vi "mod_Create Continuous FSK (generic PN).vi"(0 "Filter Length":i32=8, 2 "Symbol Rate, Hz":dbl=1500000.0 format="%.2p", 4 "TX Filter":T1(ring), 6 "BT":dbl=0.5 format="%.2f", 7 "tolerance":dbl=1e-09, 8 "error in (no error)":errorcluster, 9 "bits per symbol":i32=1, 10 "PN Sequence Order":i32=9, 11 "FSK system parameters":T2={"samples per symbol (16)"=16, "symbol map"=[-650000.0, 650000.0], "symbol phase continuity"=enum."continuous"} {"symbol map" format="%.2p"}) -> (1 "error out":errorcluster={"status"=TRUE, "code"=-21816, "source"="mod_Create Continuous FSK (Bose).vi -> MT Generate Filter Coefficients.vi\r\n"}, 3 "samples per symbol":i32, 5 "output complex waveform":T3 {"Y" format="%.3f"; "dt" format="%^.2e"; "t0" format="%.4f"})   [LabVIEW 2020, in "niDMT.lvlib"]
uses:
  <vilib>/addons/Modulation/niDMT.lvlib
  <vilib>/addons/Modulation/Analog/controls/Complex Data Waveform.ctl
  <vilib>/addons/Modulation/Digital/Support/Controls/FSK System Parameters.ctl
  <vilib>/addons/Modulation/Digital/General/MT Generate Bits (Galois, PN Order).vi
  <vilib>/addons/Modulation/Digital/Support/Common/Validators/mod_Generate Bits Validate.vi
  <vilib>/addons/Modulation/Analog/support/mod_Set Error Source.vi
  <vilib>/addons/Modulation/Digital/Support/Common/Validators/mod_Generate Filter Coefficients Validate.vi
  <vilib>/addons/Modulation/Digital/General/subVIs/mod_Generate Filter Coefficients.vi
  <vilib>/addons/Modulation/Digital/General/subVIs/mod_Generate Bits PN Sequence.vi
  <vilib>/addons/Modulation/niAMT.lvlib
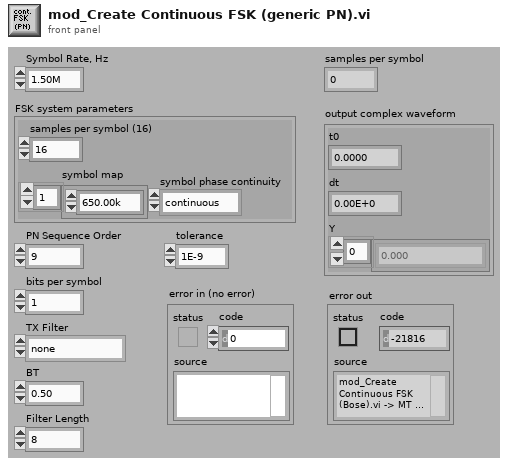
[diagram p1: front panel]
types:
  T1 = enum16{"none", "Raised Cosine", "Root Raised Cos", "Gaussian"}
  T2 = typedef "niDMT.lvlib/FSK System Parameters.ctl" = cluster{"samples per symbol (16)":i32, "symbol map":dbl[], "symbol phase continuity":enum16{"continuous", "discontinuous"}}
  T3 = typedef "niAMT.lvlib/Complex Data Waveform.ctl" = cluster{"t0":dbl, "dt":dbl, "Y":cdb[]}
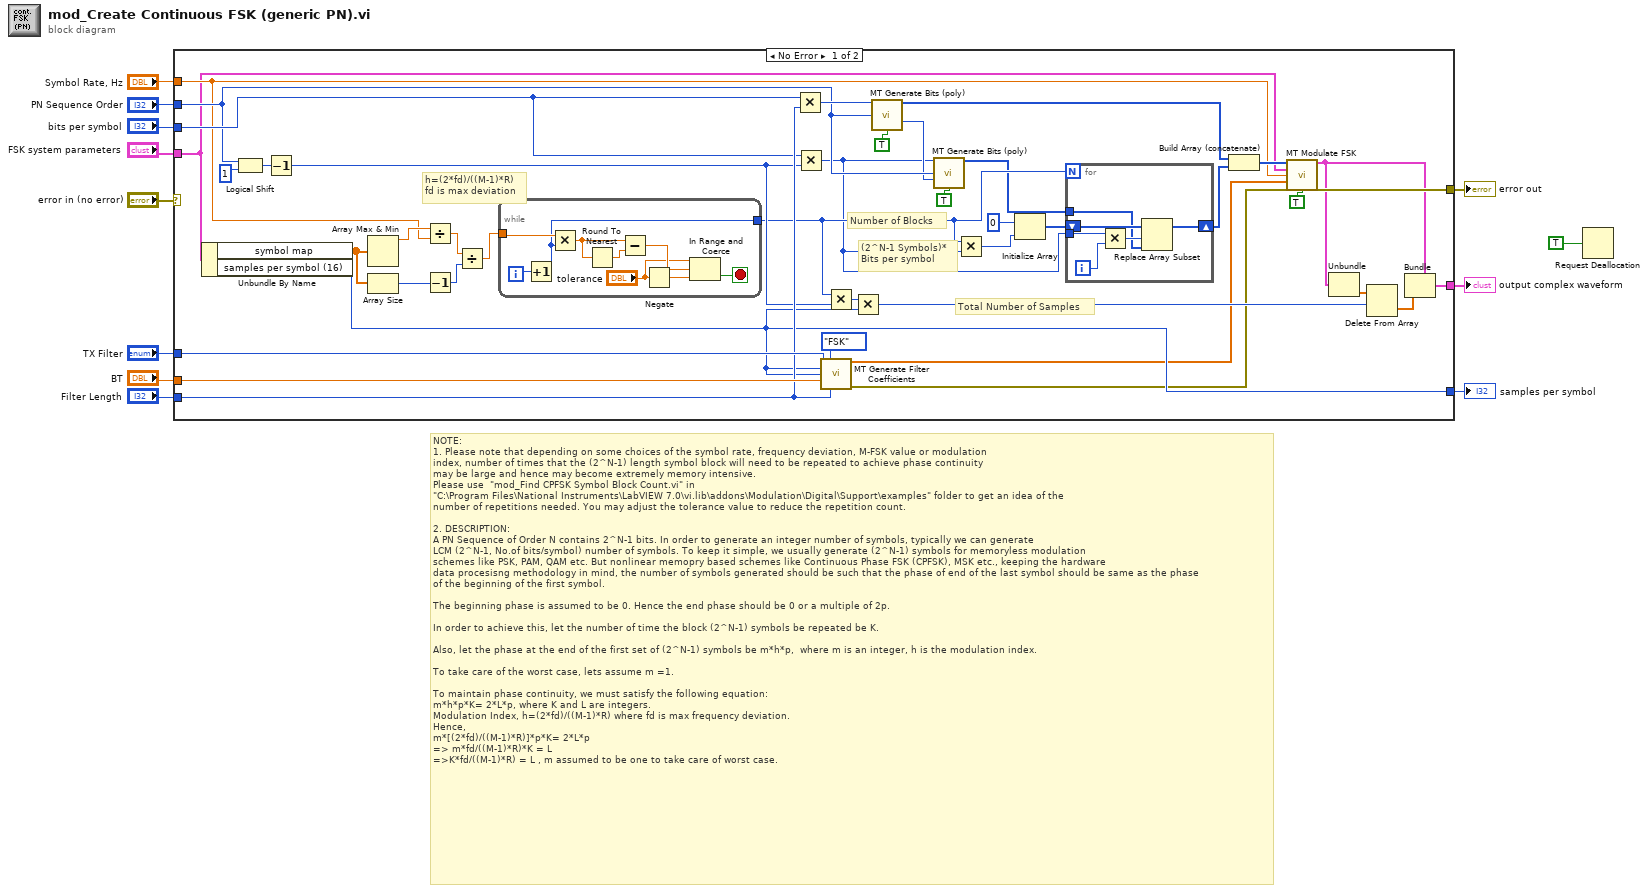
[diagram p0: block diagram]
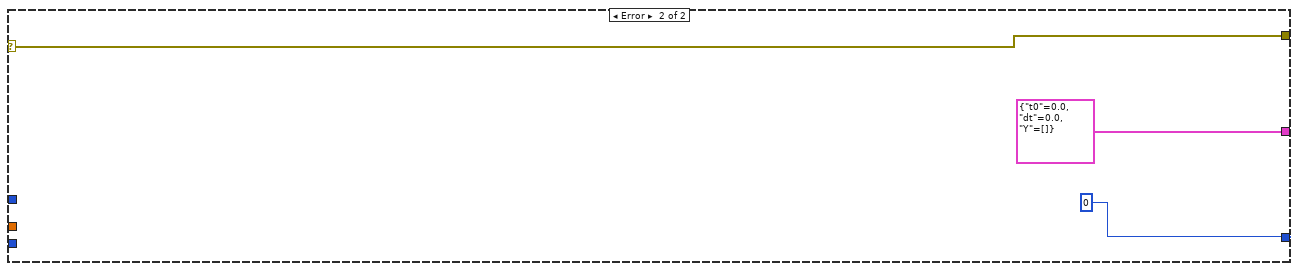
[diagram p2: hidden frame]
diagram:
  # "NOTE:\n1. Please note that depending on some choices of the symbol rate, frequency deviation, M-FSK value or modulation \nindex, number of times that the (2^N-1) length symbol block will need to be repeated to achieve phase continuity \nmay be large and hence may become extremely memory intensive. \nPlease use  \"mod_Find CPFSK Symbol Block Count.vi\" in  \n\"C:\\Program Files\\National Instruments\\LabVIEW 7.0\\vi.lib\\addons\\Modulation\\Digital\\Support\\examples\" folder to get an idea of the \nnumber of repetitions needed. You may adjust the tolerance value to reduce the repetition count.\n\n2. DESCRIPTION: \nA PN Sequence of Order N contains 2^N-1 bits. In order to generate an integer number of symbols, typically we can generate \nLCM (2^N-1, No.of bits/symbol) number of symbols. To keep it simple, we usually generate (2^N-1) symbols for memoryless modulation \nschemes like PSK, PAM, QAM etc. But nonlinear memopry based schemes like Continuous Phase FSK (CPFSK), MSK etc., keeping the hardware \ndata procesisng methodology in mind, the number of symbols generated should be such that the phase of end of the last symbol should be same as the phase \nof the beginning of the first symbol. \n\nThe beginning phase is assumed to be 0. Hence the end phase should be 0 or a multiple of 2p. \n\nIn order to achieve this, let the number of time the block (2^N-1) symbols be repeated be K. \n\nAlso, let the phase at the end of the first set of (2^N-1) symbols be m*h*p,  where m is an integer, h is the modulation index. \n\nTo take care of the worst case, lets assume m =1. \n\nTo maintain phase continuity, we must satisfy the following equation: \nm*h*p*K= 2*L*p, where K and L are integers. \nModulation Index, h=(2*fd)/((M-1)*R) where fd is max frequency deviation. \nHence, \nm*[(2*fd)/((M-1)*R)]*p*K= 2*L*p \n=> m*fd/((M-1)*R)*K = L \n=>K*fd/((M-1)*R) = L , m assumed to be one to take care of worst case."
  n1 = case shown="No Error" "error in (no error)" {
    selector: "error in (no error)" -> [_ w69]
    tunnel: [w53 w69] -> w12
    tunnel: [w52 cluster{"t0":dbl, "dt":dbl, "Y":cdb[]} {"t0"=0.0, "dt"=0.0, "Y"=[]} ("output complex waveform")] -> w10
    tunnel: [w31 0 ("samples per symbol (16)")] -> w9
    tunnel: "Symbol Rate, Hz" -> [w16 _]
    tunnel: "PN Sequence Order" -> [w24 _]
    tunnel: "bits per symbol" -> [w25 _]
    tunnel: "FSK system parameters" -> [w15 _]
    tunnel: "TX Filter" -> [w38 _]
    tunnel: "BT" -> [w37 _]
    tunnel: "Filter Length" -> [w36 _]
    frame No Error {
      # "Total Number of Samples"
      # "Number of Blocks"
      # "(2^N-1 Symbols)*\nBits per symbol"
      # "h=(2*fd)/((M-1)*R)\nfd is max deviation"
      n2 = Unbundle By Name(w15) -> ("symbol map"=w30:dbl[], "samples per symbol (16)"=w31:i32)
      n3 = Logical Shift(y=w24, x=1) -> (x << y=w46:i32)
      n4 = Decrement(x=w46) -> (x-1=w33:i32)
      n5 = Array Max & Min(array=w30) -> (max value=w29:dbl)  [unwired: 3 out]
      n6 = Array Size(array=w30) -> (size(s)=w34:i32)
      n7 = Divide(x=w29, y=w16) -> (x/y=w28:dbl)
      n8 = Decrement(x=w34) -> (x-1=w27:i32)
      n9 = Divide(x=w28, y=w27) -> (x/y=w26:dbl)
      n10 = while {
        tunnel: w26 -> [w61]
        tunnel: [w54] -> w22
        i -> [w62]
        stop <- w56 stop-if-true
        n11 = Increment(x=w62) -> (x+1=w54:i32)
        n12 = Multiply(x=w61, y=w54) -> (x*y=w55:dbl)
        n13 = Round To Nearest(number=w55) -> (nearest integer value=w60:dbl)
        n14 = Subtract(x=w55, y=w60) -> (x-y=w59:dbl)
        n15 = Negate(x="tolerance") -> (-x=w57:dbl)
        n16 = In Range and Coerce(upper limit="tolerance", x=w59, lower limit=w57) -> (In Range?=w56:bool)  [unwired: 1 out]
      }
      n17 = Multiply(x=w25, y=w36) -> (x*y=w49:i32)
      n18 = Multiply(x=w25, y=w33) -> (x*y=w20:i32)
      n19 = call <vilib>:"MT Generate Filter Coefficients.vi"("pulse shaping filter (none)"=w38, "modulation type"=enum16{"FSK", "PSK", "QAM", "MSK"}."FSK" ("Modulation Type"), "pulse shaping samples per symbol (16)"=w31, "matched samples per symbol (16)"=w31, "filter parameter"=w37, "filter length (symbols)"=w36) -> ("pulse shaping filter coefficients"=w17:dbl[], "error out"=w14:errorcluster)  [unwired: 1 in, 7 out]
      n20 = Multiply(x=w22, y=w33) -> (x*y=w32:i32)
      n21 = Multiply(x=w32, y=w31) -> (x*y=w35:i32)
      n22 = call-poly <vilib>:"MT Generate Bits (poly).vi"("total bits (128)"=w49, "PN sequence order (9)"=w24, "reset? (T)"=TRUE ("Reset (T)")) -> ("output bit stream"=w19:i8[], "seed out"=w23:i32)  [unwired: 2 in, 9 out]
      n23 = call-poly <vilib>:"MT Generate Bits (poly).vi"("total bits (128)"=w20, "PN sequence order (9)"=w24, "seed in (0xD6BF7DF2)"=w23, "reset? (T)"=TRUE ("Reset (T)")) -> ("output bit stream"=w21:i8[])  [unwired: 1 in, 10 out]
      n24 = Multiply(x=w22, y=w20) -> (x*y=w41:i32)
      n25 = Initialize Array(i8 0 ("element"), w41) -> (w42:i8[])
      n26 = for {
        N: w22 -> [_]
        shift-right: [w67] -> w18
        shift-left: w42 -> [w68]
        tunnel: w20 -> [w65]
        tunnel: w21 -> [w63]
        i -> [w66]
        n27 = Multiply(x=w65, y=w66) -> (x*y=w64:i32)
        n28 = Replace Array Subset(array=w68, new element=w63, index=w64) -> (w67:i8[])
      }
      n29 = Build Array (concatenate)(w19, w18) -> (w40:i8[])
      n30 = call <vilib>:"MT Modulate FSK.vi"("input bit stream"=w40, "FSK system parameters"=w15, "symbol rate (Hz)"=w16, "pulse shaping filter coefficients"=w17, "error in (no error)"=w14, "reset? (T)"=TRUE ("Reset (T)")) -> ("output complex waveform"=w13:T3, "error out"=w53:errorcluster)  [unwired: 1 in, 7 out]
      n31 = Unbundle(w13) -> ("Y"=w39:cdb[])  [unwired: 2 out]
      n32 = Delete From Array(array=w39, length=w35) -> (deleted portion=w51:cdb[])  [unwired: 1 in, 1 out]
      n33 = Bundle(cluster=w13, "Y"=w51) -> (w52:T3)  [unwired: 2 out]
    }
    frame Error {
    }
  }
  "error out" <- w12
  "output complex waveform" <- w10
  "samples per symbol" <- w9
  n34 = Request Deallocation(TRUE ("flag")) -> ()
